vi "Easy Hilbert Expansion.vi"(8 "error in (no error)":errorcluster, 11 "RefNum in":T1) -> (0 "error out":errorcluster, 2 "time waveform":dbl[](array[numeric]) format="%.2f", 3 "RefNum out":T1)   [LabVIEW 2017, in "SoundVib_Gabor.lvlib"]
doc: "Performs a simplified Gabor expansion on the Gabor coefficients pointed to by <B>RefNum in</B> and returns the resulting 1D time waveform in <B>time waveform</B>."
uses:
  <vilib>/addons/Sound and Vibration/Order Analysis/Gabor Order Tracking/SoundVib_Gabor.lvlib
  <vilib>/addons/Sound and Vibration/Order Analysis/Ref Gabor Order Tracking/GT RefNum.ctl
  <resource>/sndvib.dll
panel:
  # "Easy Hilbert Expansion"
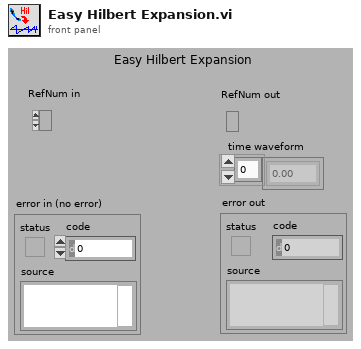
[diagram p1: front panel]
types:
  T1 = typedef "SoundVib_Gabor.lvlib/GT RefNum.ctl" = refnum<k1>
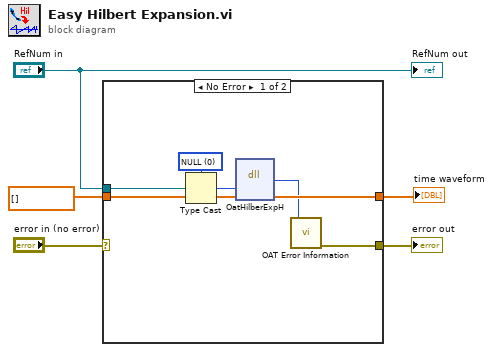
[diagram p0: block diagram]
diagram:
  n1 = case shown="No Error" "error in (no error)" {
    selector: "error in (no error)" -> [_ w14]
    tunnel: [w12 w14] -> w5
    tunnel: "RefNum in" -> [w10 _]
    tunnel: [w11 w13] -> w2
    tunnel: dbl[] [] ("Time Series") -> [w6 w13]
    frame No Error {
      w9 = u32 0 items=["NULL"]
      n2 = Type Cast(type=w9, x=w10) -> (*(type *) &x=w8:u32)
      n3 = dll-call lib="C:/Program Files (x86)/National Instruments/LabVIEW 2017/resource/sndvib.*" fn="OatHilberExpH"("refIn"=w8, "Time Series"=w6) -> ("return type"=w7:i32, "Time Series"=w11:dbl[])  [unwired: 4 in, 2 out]
      n4 = call <vilib>:"OAT Error Information.vi"("error code"=w7) -> ("error out"=w12:errorcluster)  [unwired: 6 in]
    }
    frame Error {
    }
  }
  "error out" <- w5
  "time waveform" <- w2
  "RefNum out" <- "RefNum in"
